vi "Write Element of Weight Slots.vi"(8 "error in (no error)":errorcluster, 9 "Weight Slot":T1, 10 "index":i32, 11 "WorkTable Class in":refnum<class "WorkTable Class.lvclass">) -> (0 "error out":errorcluster, 3 "WorkTable Class out":refnum<class "WorkTable Class.lvclass">)   [LabVIEW 2011, in "WorkTable Class.lvclass"]
uses:
  WorkTable Class.lvclass
  WorkTable Class.lvclass/WorkTable Class.ctl
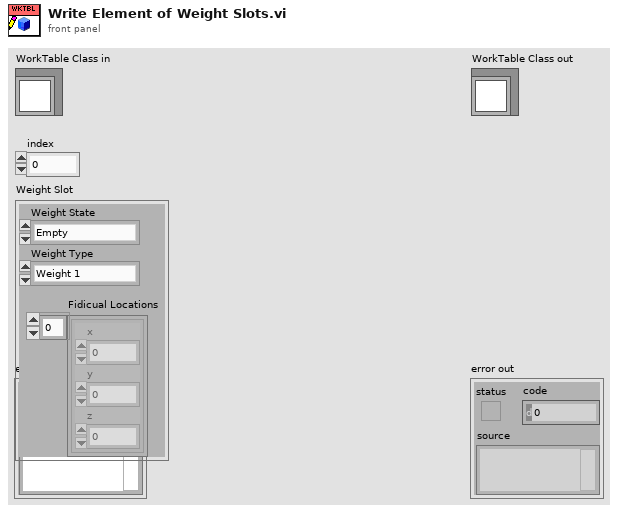
[diagram p1: front panel]
types:
  T1 = cluster{"Weight State":enum16{"Empty", "Populated"}, "Weight Type":enum16{"Weight 1", "Weight 2", "Weight 3", "Weight 4"}, "Fidicual Locations":cluster{"x":dbl, "y":dbl, "z":dbl}[]}
  T2 = cluster{"Weight State":enum16{"Empty", "Populated"}, "Weight Type":enum16{"Weight 1", "Weight 2", "Weight 3", "Weight 4"}, "Fidicual Locations":cluster{"x":dbl, "y":dbl, "z":dbl}[]}[]
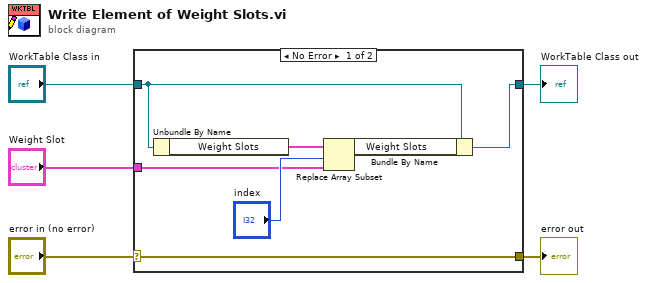
[diagram p0: block diagram]
diagram:
  n1 = case shown="No Error" "error in (no error)" {
    selector: "error in (no error)" -> [w12 w13]
    tunnel: [w12 w13] -> w4
    tunnel: [w11 w14] -> w2
    tunnel: "WorkTable Class in" -> [w10 w14]
    tunnel: "Weight Slot" -> [w6 _]
    frame No Error {
      n2 = Unbundle By Name(w10) -> ("Weight Slots"=w9:T2)
      n3 = Replace Array Subset(array=w9, new element=w6, index="index") -> (w8:T2)
      n4 = Bundle By Name(cluster=w10, "Weight Slots"=w8) -> (w11:refnum<class "WorkTable Class.lvclass">)
    }
    frame Error {
    }
  }
  "error out" <- w4
  "WorkTable Class out" <- w2
